vi "_Read_Z.vi"(8 "error in (no error)":errorcluster, 11 "Postgres Connector In":refnum<class "Postgres Connector.lvclass">) -> (0 "error out":errorcluster, 2 "State After Query":string, 3 "Postgres Connector Out":refnum<class "Postgres Connector.lvclass">)   [LabVIEW 2020, in "Postgres Connector.lvclass"]
doc: "This VI return the status of the database at the end of a query.s"
uses:
  Postgres Connector.lvclass
  Cluster_Reader_Infos.ctl
  Postgres Connector.lvclass/Postgres Connector.ctl
  Enum_RowDescription_State_Machine.ctl
panel:
  out "data out":string
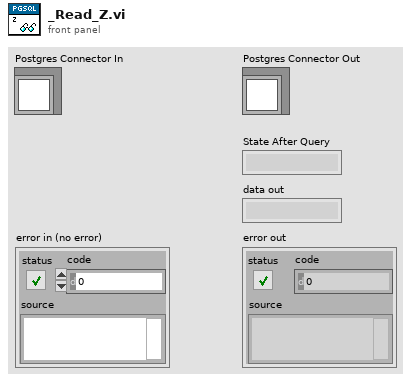
[diagram p1: front panel]
types:
  T1 = typedef "Postgres Connector.lvclass/Cluster_Reader_Infos.ctl" = cluster{"Byte Length":i32}
  T2 = typedef "Postgres Connector.lvclass/Enum_RowDescription_State_Machine.ctl" = enum16{"Check For Error", "Wait For T", "Wait For D", "Wait For Z", "C Byte Length", "Z Byte Length", "n Byte Length", "Byte Length", "Get Infos", "Check For End", "Flush", "Quit"}
  T3 = enum16{"Standard", "Buffered", "CRLF", "Immediate"}
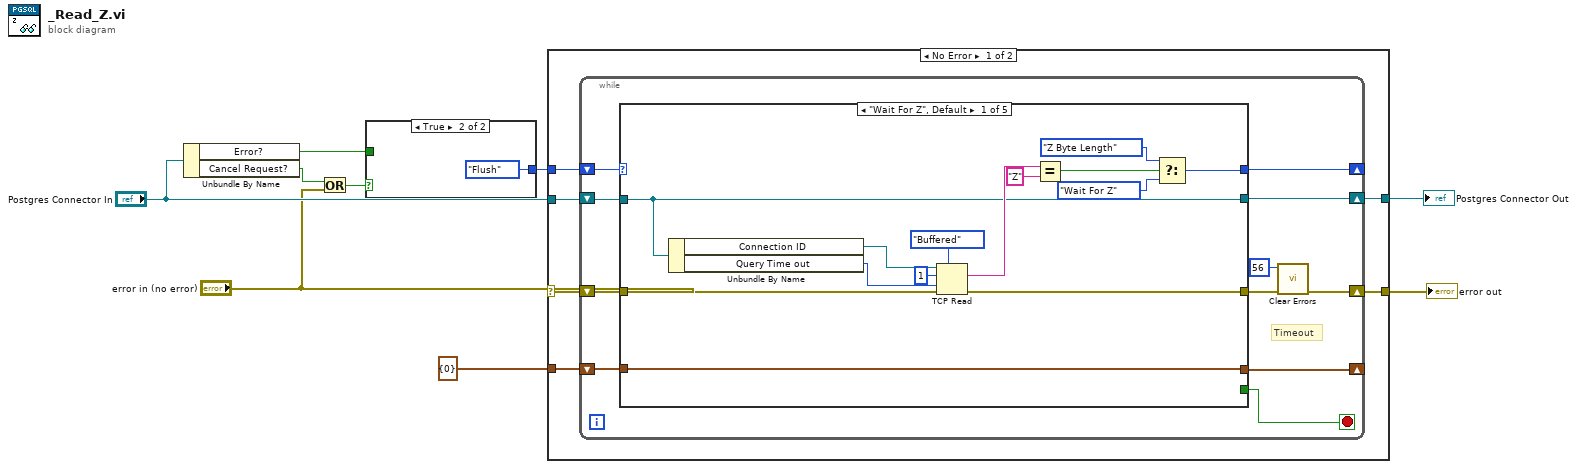
[diagram p0: block diagram]
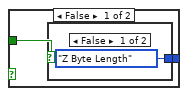
[diagram p2: hidden frame]
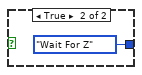
[diagram p3: hidden frame]
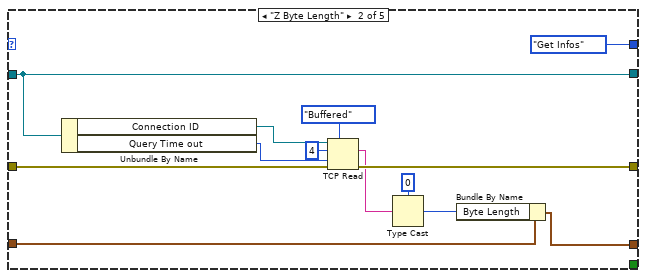
[diagram p4: hidden frame]
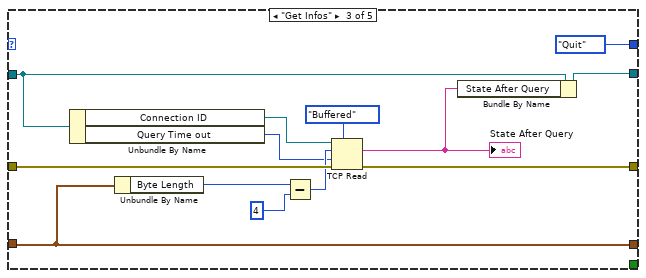
[diagram p5: hidden frame]
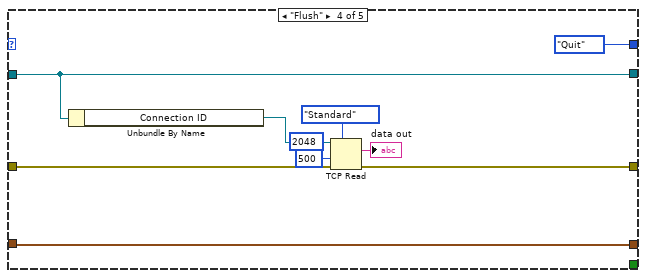
[diagram p6: hidden frame]
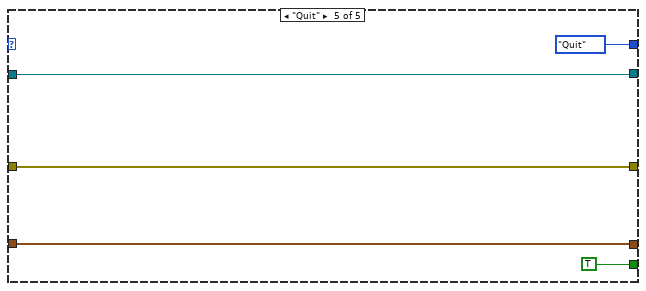
[diagram p7: hidden frame]
diagram:
  n1 = Unbundle By Name("Postgres Connector In") -> ("Error?"=w5:bool, "Cancel Request?"=w2:bool)
  n2 = Or(x=w2, y="error in (no error)") -> (x .or. y?=w1:bool)
  n3 = case shown="True" w1 {
    tunnel: [w11 Enum_RowDescription_State_Machine."Flush"] -> w9
    tunnel: w5 -> [w10 _]
    frame False {
      n4 = case shown="False" w10 {
        tunnel: [Enum_RowDescription_State_Machine."Z Byte Length" Enum_RowDescription_State_Machine."Wait For Z"] -> w11
        frame False {
        }
        frame True {
        }
      }
    }
    frame True {
    }
  }
  n5 = case shown="No Error" "error in (no error)" {
    selector: "error in (no error)" -> [w19 w88]
    tunnel: "Postgres Connector In" -> [w20 w87]
    tunnel: w9 -> [w18 _]
    tunnel: [w17 w88] -> w8
    tunnel: T1 {"Byte Length"=0} ("Reader_Infos") -> [w16 _]
    tunnel: [w15 w87] -> w4
    frame No Error {
      n6 = while {
        shift-right: [w27] -> w17
        shift-left: w19 -> [w30]
        shift-right: [w25] -> _
        shift-left: w18 -> [w29]
        shift-right: [w23] -> _
        shift-left: w16 -> [w24]
        shift-right: [w21] -> w15
        shift-left: w20 -> [w31]
        stop <- w22 stop-if-true
        # "Timeout"
        n7 = case shown="\"Wait For Z\", Default" w29 {
          tunnel: w31 -> [w40 w55 w62 w78 w82]
          tunnel: w30 -> [w41 w54 w69 w77 w85]
          tunnel: [w39 w53 w68 w74 w85] -> w28
          tunnel: [w36 Enum_RowDescription_State_Machine."Get Infos" Enum_RowDescription_State_Machine."Quit" Enum_RowDescription_State_Machine."Quit" Enum_RowDescription_State_Machine."Quit"] -> w25
          tunnel: w24 -> [w33 w51 w66 w76 w86]
          tunnel: [w33 w50 w66 w76 w86] -> w23
          tunnel: [_ _ _ _ TRUE] -> w22
          tunnel: [w40 w55 w60 w78 w82] -> w21
          frame "Wait For Z", Default {
            n8 = Unbundle By Name(w40) -> ("Connection ID"=w44:refnum<k5>, "Query Time out"=w32:i32)
            n9 = TCP Read(connection ID=w44, bytes to read=1, error in (no error)=w41, 7:T3."Buffered" ("mode (standard)"), 9:w32) -> (data out=w42:string, error out=w39:errorcluster)  [unwired: 1 out]
            n10 = Equal?(x=w42, y="Z") -> (x = y?=w37:bool)
            n11 = Select(t=Enum_RowDescription_State_Machine."Z Byte Length", s=w37, f=Enum_RowDescription_State_Machine."Wait For Z") -> (s? t:f=w36:T2)
          }
          frame "Z Byte Length" {
            n12 = Unbundle By Name(w55) -> ("Connection ID"=w57:refnum<k5>, "Query Time out"=w46:i32)
            n13 = TCP Read(connection ID=w57, bytes to read=4, error in (no error)=w54, 7:T3."Buffered" ("mode (standard)"), 9:w46) -> (data out=w47:string, error out=w53:errorcluster)  [unwired: 1 out]
            n14 = Type Cast(type=0, x=w47) -> (*(type *) &x=w48:i32)
            n15 = Bundle By Name(cluster=w51, "Byte Length"=w48) -> (w50:T1)
          }
          frame "Get Infos" {
            n16 = Unbundle By Name(w62) -> ("Connection ID"=w70:refnum<k5>, "Query Time out"=w59:i32)
            n17 = Unbundle By Name(w66) -> ("Byte Length"=w65:i32)
            n18 = Subtract(x=w65, y=4 ("bytes to read")) -> (x-y=w64:i32)
            n19 = TCP Read(connection ID=w70, bytes to read=w64, error in (no error)=w69, 7:T3."Buffered" ("mode (standard)"), 9:w59) -> (data out=w61:string, error out=w68:errorcluster)  [unwired: 1 out]
            "State After Query" <- w61
            n20 = Bundle By Name(cluster=w62, "State After Query"=w61) -> (w60:refnum<class "Postgres Connector.lvclass">)
          }
          frame "Flush" {
            n21 = Unbundle By Name(w78) -> ("Connection ID"=w80:refnum<k5>)
            n22 = TCP Read(connection ID=w80, bytes to read=2048, error in (no error)=w77, 7:T3."Standard" ("mode (standard)"), 9:500 ("timeout ms (25000)")) -> (data out=→"data out":string, error out=w74:errorcluster)  [unwired: 1 out]
          }
          frame "Quit" {
          }
        }
        n23 = call <vilib>:"Clear Errors.vi"("error in (no error)"=w28, "specific error code to clear (0: all)"=56) -> ("error out"=w27:errorcluster)  [unwired: 4 in, 1 out]
      }
    }
    frame Error {
    }
  }
  "error out" <- w8
  "Postgres Connector Out" <- w4
